vi "Flatness_1.vi"() -> ()   [LabVIEW 2020]
uses:
  Support/Controls/Cmd_Mouse Popup.ctl
  Support/Controls/Clst_Initialize Input.ctl
  Support/Controls/Cmd_Var Data IO.ctl
  Support/Controls/Cmd_STD select.ctl
  Variables/Global_Cal Info.vi
  Variables/Global_Cal STD.vi
panel:
  out "기준기분해능 (μm)":string
  in  "기준기 설정":string(combo)
  in  "Spec 변경":bool
  in  "Random":bool
  out "Spec":string[][](table)
  out "제목":string
  out "에러 출력":errorcluster
  out "Condition":string[][](table) caption="2. 직선성 시험"
  in  "Measured":string[][](table) caption="기준기 지시값 (μm)"
  out "Load?":bool
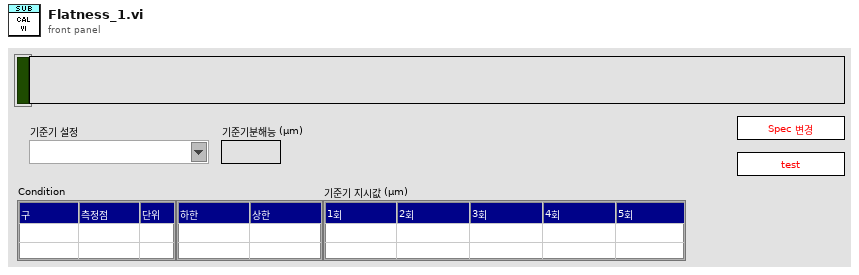
[diagram p1: front panel]
types:
  T1 = typedef "Cmd_Mouse Popup.ctl" = enum16{"활성화", "메뉴선택"}
  T2 = cluster{"Shift":bool, "Ctrl":bool, "Alt":bool, "Cmd":bool, "Opt":bool}
  T3 = typedef "Clst_Initialize Input.ctl" = cluster{"Initialize 1":cluster{"Condition":refnum<vi>[], "Spec":refnum<vi>[], "Measured":refnum<vi>[], "Resolution":refnum<vi>[], "Func_ext":string, "제목":refnum<vi>, "Measured_ADJ":refnum<vi>[]}, "Initialize 2":cluster{"문자열":refnum<vi>[], "콤보박스":refnum<vi>[], "링":refnum<vi>[], "열거형":refnum<vi>[], "테이블":refnum<vi>[], "여러열":refnum<vi>[], "디지털(DBL)":refnum<vi>[], "3D string":refnum<vi>[], "ctrl":refnum<vi>[], "boolean":refnum<vi>[]}}
  T4 = typedef "Cmd_Var Data IO.ctl" = enum16{"Condition", "Condition Default", "Condition_Temp", "Resolution", "Resolution Default", "Resolution Old", "Spec", "Spec Default", "Spec Old", "Spec Temp", "Result", "Result2", "Result3", "Result_Temp", "Result_ADJ", "Result_ADJ2", "STD1", "STD2", "STD3", "STD4", "STD5", "STD Temp", "CMC", "CMC Default"}
  T5 = typedef "Cmd_STD select.ctl" = enum16{"기본", "DMM", "Electronic Micrometer", "Fine Angle Generator", "Measuring Projector", "Precision Square", "Power Supply", "Ring Gauge", "Straight Edge", "Thermo-Hygrometer", "Calibrator"}
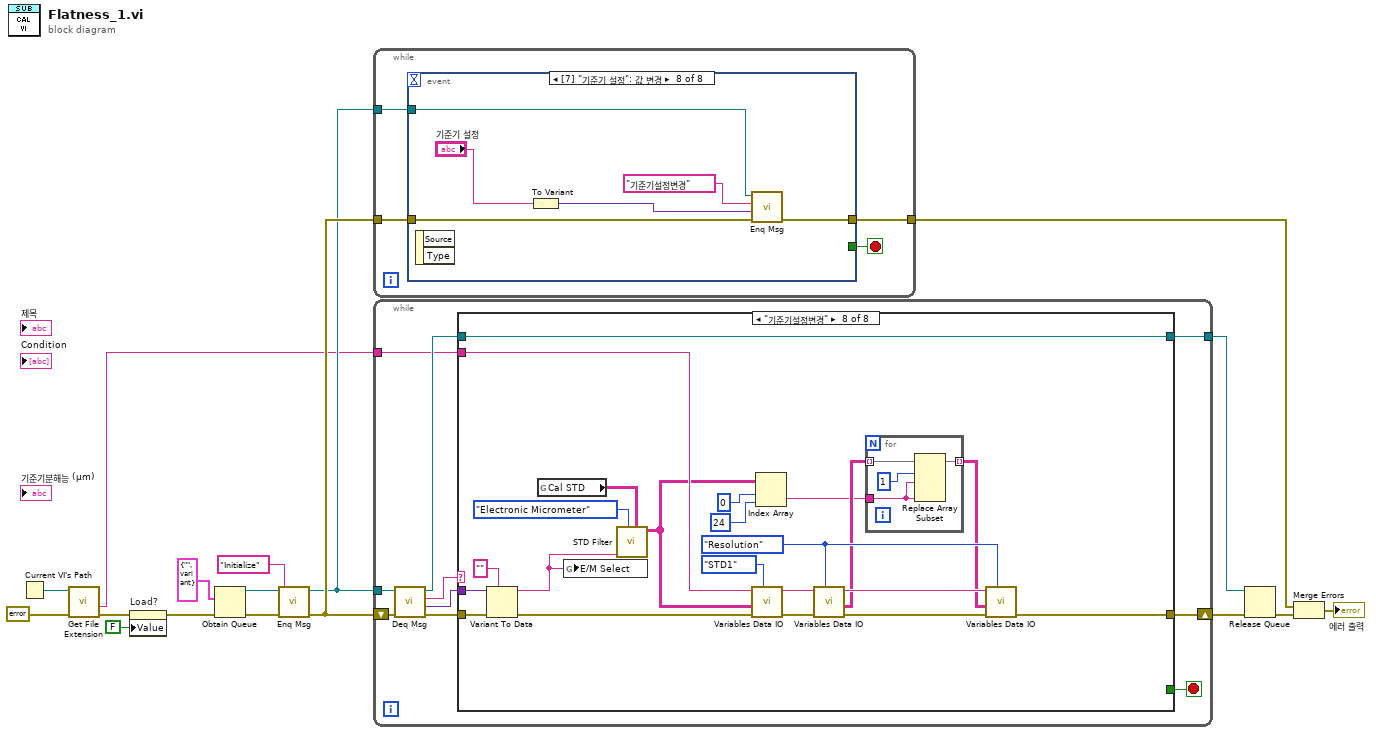
[diagram p0: block diagram]
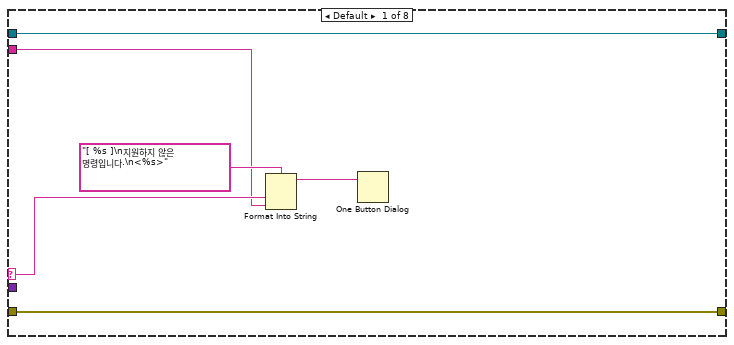
[diagram p2: hidden frame]
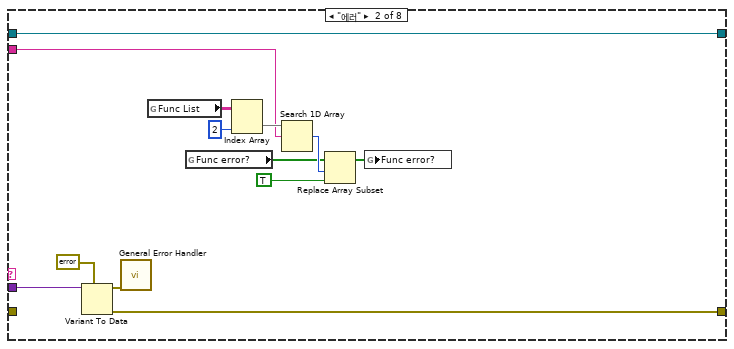
[diagram p3: hidden frame]
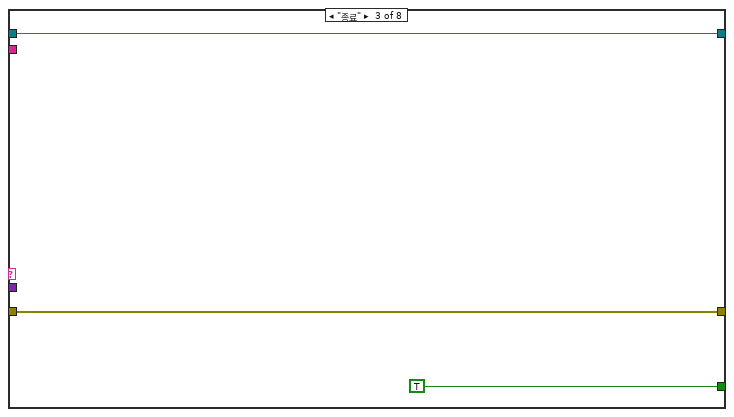
[diagram p4: hidden frame]
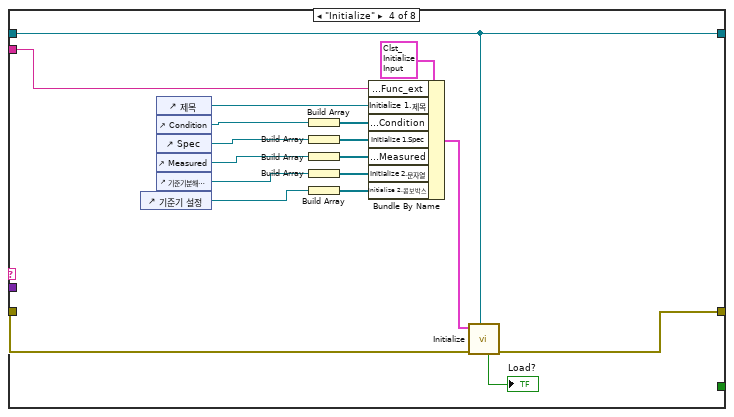
[diagram p5: hidden frame]
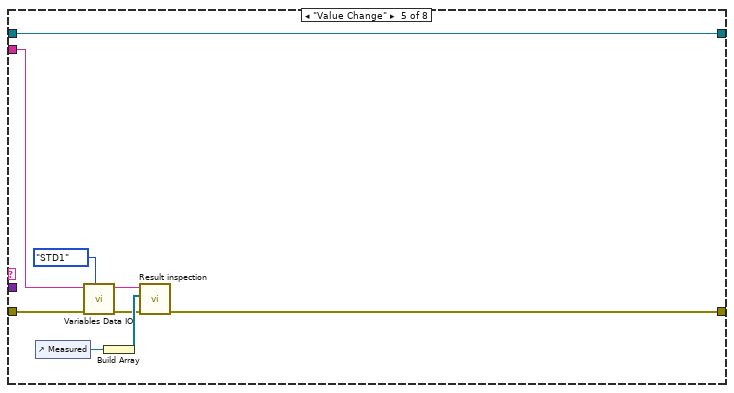
[diagram p6: hidden frame]
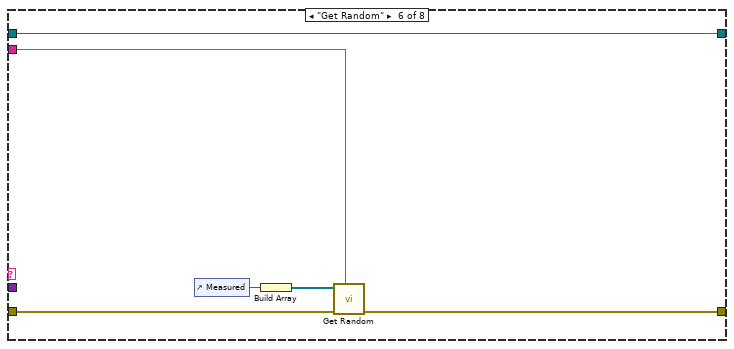
[diagram p7: hidden frame]
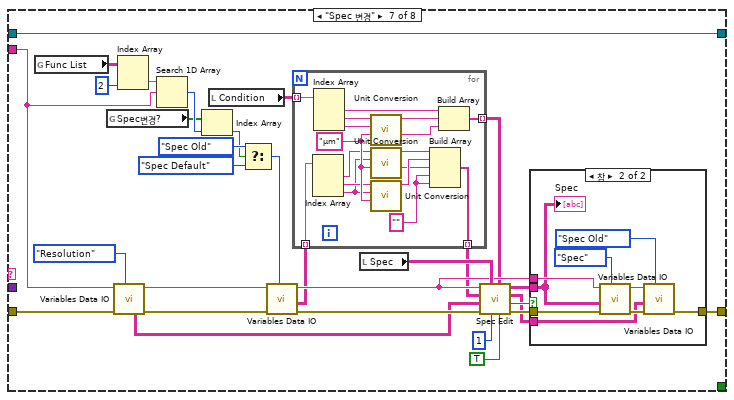
[diagram p8: hidden frame]
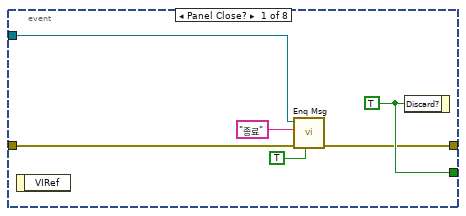
[diagram p10: hidden frame]
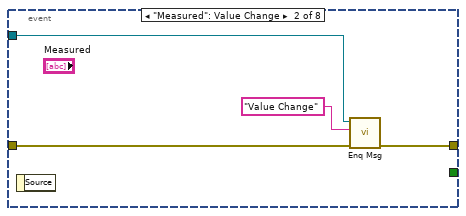
[diagram p11: hidden frame]
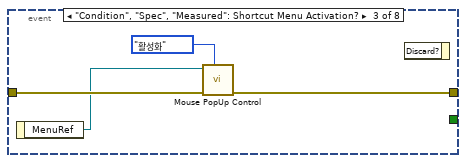
[diagram p12: hidden frame]
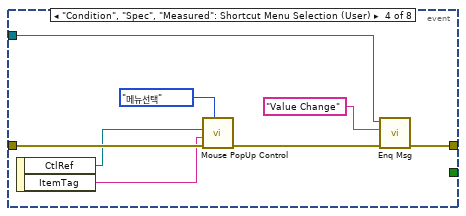
[diagram p13: hidden frame]
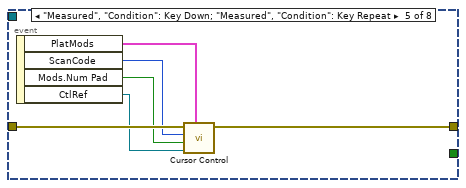
[diagram p14: hidden frame]
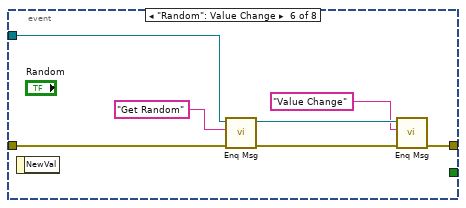
[diagram p15: hidden frame]
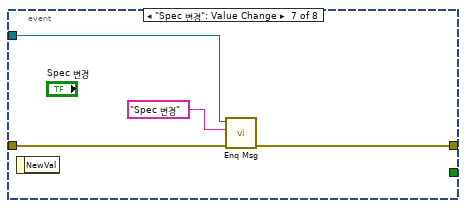
[diagram p16: hidden frame]
diagram:
  n1 = Current VI's Path() -> (path=w5:path)
  n2 = call <vilib>:"Get File Extension.vi"("error in (no error)"=errorcluster {"status"=FALSE, "code"=0, "source"=""} ("에러 상수"), "file"=w5) -> ("error out"=w3:errorcluster, "filename without extension"=w4:string)  [unwired: 5 in, 3 out]
  n3 = property on="Load?" class="Bool (엄격한)"(error in=w3, "Value"=FALSE ("Load?")) -> (error out=w2:errorcluster)  [unwired: 1 in, 1 out]
  n4 = Obtain Queue(element data type=cluster{"메세지":string, "값":variant} {"메세지"="", "값"=variant} ("Message Cluster"), error in (no error)=w2) -> (queue out=w14:refnum<queue>, error out=w16:errorcluster)  [unwired: 3 in, 1 out]
  n5 = call "Enq Msg.vi"("에러 입력(에러 없음)"=w16, "메세지"="Initialize", "큐 입력"=w14) -> ("에러 출력"=w15:errorcluster, "큐 출력"=w12:refnum<queue>)  [unwired: 7 in]
  n6 = while {
    tunnel: w15 -> [w19]
    tunnel: w12 -> [w20]
    tunnel: [w18] -> w9
    stop <- w21 stop-if-true
    n7 = event shown="[7] \"기준기 설정\": 값 변경" {
      selector: _ -> [_ _ _ _ _ _ _ _]
      dyn-events: _ -> [_ _ _ _ _ _ _ _]
      timeout: _ -> [_ _ _ _ _ _ _ _]
      tunnel: [w27 _ _ _ _ _ _ _] -> w21
      tunnel: w20 -> [w25 w31 _ w36 _ w54 w58 w63]
      tunnel: w19 -> [w26 w29 w35 w43 w49 w55 w59 w65]
      tunnel: [w23 w30 w34 w37 w48 w50 w57 w64] -> w18
      event Panel Close? {
        w27 = TRUE ("버림?")
        n8 = event-data() -> ()  [unwired: 1 in, 1 out]
        n9 = call "Enq Msg.vi"("우선순위 메시지?"=TRUE, "에러 입력(에러 없음)"=w26, "메세지"="종료", "큐 입력"=w25) -> ("에러 출력"=w23:errorcluster)  [unwired: 6 in, 1 out]
        n10 = event-data("Discard?"=w27) -> ()  [unwired: 1 in, 1 out]
      }
      event "Measured": Value Change {
        n11 = event-data() -> ()  [unwired: 1 in, 1 out]
        n12 = call "Enq Msg.vi"("에러 입력(에러 없음)"=w29, "메세지"="Value Change", "큐 입력"=w31) -> ("에러 출력"=w30:errorcluster)  [unwired: 7 in, 1 out]
      }
      event "Condition", "Spec", "Measured": Shortcut Menu Activation? {
        n13 = event-data() -> ("MenuRef"=w33:refnum<k9>)  [unwired: 1 in]
        n14 = call "Mouse PopUp Control.vi"("type"=Cmd_Mouse_Popup."활성화", "error in"=w35, "메뉴 참조"=w33) -> ("error out"=w34:errorcluster)  [unwired: 8 in]
        n15 = event-data() -> ()  [unwired: 2 in, 1 out]
      }
      event "Condition", "Spec", "Measured": Shortcut Menu Selection (User) {
        n16 = event-data() -> ("CtlRef"=w41:refnum<vi>, "ItemTag"=w40:string)  [unwired: 1 in]
        n17 = call "Mouse PopUp Control.vi"("type"=Cmd_Mouse_Popup."메뉴선택", "error in"=w43, "아이템 태그"=w40, "Tbl 참조 번호"=w41) -> ("error out"=w38:errorcluster)  [unwired: 7 in]
        n18 = call "Enq Msg.vi"("에러 입력(에러 없음)"=w38, "메세지"="Value Change", "큐 입력"=w36) -> ("에러 출력"=w37:errorcluster)  [unwired: 7 in, 1 out]
      }
      event "Measured", "Condition": Key Down; "Measured", "Condition": Key Repeat {
        n19 = event-data() -> ("PlatMods"=w44:T2, "ScanCode"=w47:i16, "Mods.Num Pad"=w46:bool, "CtlRef"=w45:refnum<vi>)  [unwired: 1 in]
        n20 = call "Cursor Control.vi"("플랫폼 조합키"=w44, "참조"=w45, "Num Pad"=w46, "ScanCode"=w47, "error in"=w49) -> ("error out"=w48:errorcluster)  [unwired: 5 in, 1 out]
      }
      event "Random": Value Change {
        n21 = event-data() -> ()  [unwired: 1 in, 1 out]
        n22 = call "Enq Msg.vi"("에러 입력(에러 없음)"=w55, "메세지"="Get Random", "큐 입력"=w54) -> ("에러 출력"=w53:errorcluster, "큐 출력"=w52:refnum<queue>)  [unwired: 7 in]
        n23 = call "Enq Msg.vi"("에러 입력(에러 없음)"=w53, "메세지"="Value Change", "큐 입력"=w52) -> ("에러 출력"=w50:errorcluster)  [unwired: 7 in, 1 out]
      }
      event "Spec 변경": Value Change {
        n24 = event-data() -> ()  [unwired: 1 in, 1 out]
        n25 = call "Enq Msg.vi"("에러 입력(에러 없음)"=w59, "메세지"="Spec 변경", "큐 입력"=w58) -> ("에러 출력"=w57:errorcluster)  [unwired: 7 in, 1 out]
      }
      event "기준기 설정": Value Change {
        n26 = event-data() -> ()  [unwired: 1 in, 2 out]
        n27 = To Variant(anything="기준기 설정") -> (Variant=w61:variant)
        n28 = call "Enq Msg.vi"("에러 입력(에러 없음)"=w65, "값"=w61, "메세지"="기준기설정변경", "큐 입력"=w63) -> ("에러 출력"=w64:errorcluster)  [unwired: 6 in, 1 out]
      }
    }
  }
  n29 = while {
    shift-right: [w76] -> w11
    shift-left: w15 -> [w75]
    tunnel: w12 -> [w73]
    tunnel: [w68] -> w10
    tunnel: w4 -> [w67]
    stop <- w69 stop-if-true
    n30 = call "Deq Msg.vi"("에러 입력(에러 없음)"=w75, "큐 입력"=w73) -> ("에러 출력"=w74:errorcluster, "값"=w70:variant, "메세지"=w72:string, "큐 출력"=w71:refnum<queue>)  [unwired: 6 in]
    n31 = case shown="\"기준기설정변경\"" w72 {
      selector: w72 -> [w78 _ _ _ _ _ _ _]
      tunnel: w74 -> [w82 _ w98 w116 w120 w127 w154 w209]
      tunnel: [w82 w92 w98 w103 w117 w128 w157 w197] -> w76
      tunnel: w71 -> [w81 w91 w96 w104 w125 w131 w161 w210]
      tunnel: w70 -> [_ w93 _ _ _ _ _ w208]
      tunnel: [_ _ TRUE ("버림?") _ _ _ _ _] -> w69
      tunnel: [w81 w91 w96 w104 w125 w131 w161 w210] -> w68
      tunnel: w67 -> [w77 w83 _ w105 w122 w126 w141 w202]
      frame Default {
        n32 = Format Into String(format string="[ %s ]\n지원하지 않은 명령입니다.\n<%s>" ("메시지"), w78, w77) -> (resulting string=w79:string)  [unwired: 2 in, 1 out]
        n33 = One Button Dialog(message=w79) -> ()  [unwired: 1 in, 1 out]
      }
      frame "에러" {
        n34 = Variant To Data(type=errorcluster {"status"=FALSE, "code"=0, "source"=""} ("에러 출력"), Variant=w93) -> (data=w95:errorcluster, error out=w92:errorcluster)  [unwired: 1 in]
        n35 = call <vilib>:"General Error Handler.vi"("error in (no error)"=w95) -> ()  [unwired: 10 in, 5 out]
        n36 = global read "Global_Cal Info.vi" "Func List"() -> (w85:string[][])
        n37 = global read "Global_Cal Info.vi" "Func error?"() -> (w88:bool[])
        n38 = Index Array(array=w85, index (col)=2 ("비활성화된 인덱스 (열)")) -> (element=w86:string[])  [unwired: 1 in]
        n39 = Search 1D Array(1D array=w86, element=w83) -> (index of element=w89:i32)  [unwired: 1 in]
        n40 = Replace Array Subset(array=w88, new element=TRUE ("새 원소/부분배열"), index=w89) -> (w90:bool[])
        n41 = global write "Global_Cal Info.vi" "Func error?"(w90) -> ()
      }
      frame "종료" {
      }
      frame "Initialize" {
        n42 = control-ref of="기준기 설정"() -> (w100:refnum<vi>)
        n43 = control-ref of="제목"() -> (w108:refnum<vi>)
        n44 = control-ref of="Condition"() -> (w113:refnum<vi>)
        n45 = control-ref of="Spec"() -> (w107:refnum<vi>)
        n46 = control-ref of="Measured"() -> (w110:refnum<vi>)
        n47 = control-ref of="기준기분해능 (μm)"() -> (w99:refnum<vi>)
        n48 = Build Array(w113) -> (w112:refnum<vi>[])
        n49 = Build Array(w107) -> (w106:refnum<vi>[])
        n50 = Build Array(w110) -> (w111:refnum<vi>[])
        n51 = Build Array(w99) -> (w109:refnum<vi>[])
        n52 = Build Array(w100) -> (w101:refnum<vi>[])
        n53 = Bundle By Name(cluster=T3 {"Initialize 1"={"Condition"=[], "Spec"=[], "Measured"=[], "Resolution"=[], "Func_ext"="", "제목"=refnum, "Measured_ADJ"=[]}, "Initialize 2"={"문자열"=[], "콤보박스"=[], "링"=[], "열거형"=[], "테이블"=[], "여러열"=[], "디지털(DBL)"=[], "3D string"=[], "ctrl"=[], "boolean"=[]}} ("입력 클러스터"), "Initialize 1.Func_ext"=w105, "Initialize 1.제목"=w108, "Initialize 1.Condition"=w112, "Initialize 1.Spec"=w106, "Initialize 1.Measured"=w111, "Initialize 2.문자열"=w109, "Initialize 2.콤보박스"=w101) -> (w114:T3)
        n54 = call "Initialize.vi"("큐 입력"=w104, "error in"=w116, "입력 클러스터"=w114) -> ("error out"=w103:errorcluster, "Load?"=→"Load?":bool)  [unwired: 5 in, 2 out]
      }
      frame "Value Change" {
        n55 = control-ref of="Measured"() -> (w124:refnum<vi>)
        n56 = call "Variables Data IO.vi"("Select"=Cmd_Var_Data_IO."STD1", "error in"=w120, "Func_ext"=w122) -> ("error out"=w118:errorcluster, "Func_ext Out"=w119:string)  [unwired: 6 in, 1 out]
        n57 = Build Array(w124) -> (w123:refnum<vi>[])
        n58 = call "Result inspection.vi"("error in"=w118, "Ref. Data (Inspection)"=w123, "Func ext"=w119) -> ("error out"=w117:errorcluster)  [unwired: 5 in, 3 out]
      }
      frame "Get Random" {
        n59 = control-ref of="Measured"() -> (w130:refnum<vi>)
        n60 = Build Array(w130) -> (w129:refnum<vi>[])
        n61 = call "Get Random.vi"("Func_Ext"=w126, "에러 입력"=w127, "Meas"=w129) -> ("에러 출력"=w128:errorcluster)  [unwired: 7 in, 1 out]
      }
      frame "Spec 변경" {
        n62 = global read "Global_Cal Info.vi" "Func List"() -> (w146:string[][])
        n63 = global read "Global_Cal Info.vi" "Spec변경?"() -> (w142:bool[])
        n64 = call "Variables Data IO.vi"("Select"=Cmd_Var_Data_IO."Resolution", "error in"=w154, "Func_ext"=w141) -> ("error out"=w139:errorcluster, "Data Out"=w137:string[][], "Func_ext Out"=w138:string)  [unwired: 6 in]
        n65 = Index Array(array=w146, index (col)=2 ("비활성화된 인덱스 (열)")) -> (element=w144:string[])  [unwired: 1 in]
        n66 = Search 1D Array(1D array=w144, element=w141) -> (index of element=w143:i32)  [unwired: 1 in]
        n67 = Index Array(array=w142, index=w143) -> (element=w147:bool)
        n68 = local read "Condition"() -> (w135:string[][])
        n69 = Select(t=Cmd_Var_Data_IO."Spec Old" ("Select"), s=w147, f=Cmd_Var_Data_IO."Spec Default" ("Select")) -> (s? t:f=w140:T4)
        n70 = call "Variables Data IO.vi"("Select"=w140, "error in"=w139, "Func_ext"=w138) -> ("error out"=w156:errorcluster, "Data Out"=w133:string[][], "Func_ext Out"=w150:string)  [unwired: 6 in]
        n71 = for {
          tunnel: w135 -> [w165] mode=indexing
          tunnel: [w166] -> w134 mode=indexing
          tunnel: w133 -> [w175] mode=indexing
          tunnel: [w168] -> w132 mode=indexing
          w167 = "" ("원소")
          w176 = "μm" ("환산단위")
          n72 = Index Array(array=w175) -> (element #1=w174:string, element #2=w173:string, element #3=w172:string)  [unwired: 3 in]
          n73 = Index Array(array=w165) -> (element #1=w164:string, element #2=w178:string, element #3=w177:string)  [unwired: 3 in]
          n74 = call "Unit Conversion.vi"("환산단위"=w176, "입력단위"=w177, "입력값"=w178) -> ("환산단위"=w162:string, "환산값 (string)"=w163:string)  [unwired: 3 in, 4 out]
          n75 = call "Unit Conversion.vi"("환산단위"=w176, "입력단위"=w172, "입력값"=w174) -> ("환산단위"=w169:string, "환산값 (string)"=w171:string)  [unwired: 3 in, 4 out]
          n76 = call "Unit Conversion.vi"("환산단위"=w176, "입력단위"=w172, "입력값"=w173) -> ("환산값 (string)"=w170:string)  [unwired: 3 in, 5 out]
          n77 = Build Array(w171, w170, w169, w167, w167) -> (w168:string[])
          n78 = Build Array(w164, w163, w162) -> (w166:string[])
        }
        n79 = local read "Spec"() -> (w151:string[][])
        n80 = call "Spec Edit.vi"("0기준?"=TRUE, "Condition"=w134, "열번호(기준값)"=1, "Spec Value"=w151, "에러 입력(에러 없음)"=w156, "Resolution"=w137, "Spec Default"=w132, "Func_ext"=w150) -> ("에러 출력"=w158:errorcluster, "변경?"=w159:bool, "Spec Default out"=w153:string[][], "Spec 출력"=w160:string[][])
        n81 = case shown="참" w159 {
          tunnel: w160 -> [_ w185]
          tunnel: w158 -> [w179 w188]
          tunnel: [w179 w183] -> w157
          tunnel: w150 -> [_ w186]
          tunnel: w153 -> [_ w181]
          frame False {
          }
          frame True {
            n82 = call "Variables Data IO.vi"("Select"=Cmd_Var_Data_IO."Spec", "error in"=w188, "Data In"=w185, "Func_ext"=w186) -> ("error out"=w184:errorcluster, "Func_ext Out"=w182:string)  [unwired: 5 in, 1 out]
            n83 = call "Variables Data IO.vi"("Select"=Cmd_Var_Data_IO."Spec Old", "error in"=w184, "Data In"=w181, "Func_ext"=w182) -> ("error out"=w183:errorcluster)  [unwired: 5 in, 2 out]
            "Spec" <- w185
          }
        }
      }
      frame "기준기설정변경" {
        w195 = Cmd_Var_Data_IO."Resolution" ("Select")
        n84 = Variant To Data(error in=w209, type="", Variant=w208) -> (data=w204:string, error out=w203:errorcluster)
        n85 = global read "Global_Cal STD.vi" "Cal STD"() -> (w205:string[][])
        n86 = global write "Global_Cal STD.vi" "E/M Select"(w204) -> ()
        n87 = call "STD Filter.vi"("Cal STD in"=w205, "STD select"=Cmd_STD_select."Electronic Micrometer", "문자열(option, STD)"=w204) -> ("DATA 출력"=w192:string[][])  [unwired: 4 in, 4 out]
        n88 = call "Variables Data IO.vi"("Select"=Cmd_Var_Data_IO."STD1", "error in"=w203, "Data In"=w192, "Func_ext"=w202) -> ("error out"=w199:errorcluster, "Func_ext Out"=w200:string)  [unwired: 5 in, 1 out]
        n89 = Index Array(array=w192, index (row)=0 ("비활성화된 인덱스 (행)"), index (col)=24 ("비활성화된 인덱스 (열)")) -> (element=w189:string)
        n90 = call "Variables Data IO.vi"("Select"=w195, "error in"=w199, "Func_ext"=w200) -> ("error out"=w198:errorcluster, "Data Out"=w194:string[][], "Func_ext Out"=w196:string)  [unwired: 6 in]
        n91 = for {
          tunnel: w194 -> [w214] mode=indexing
          tunnel: [w213] -> w193 mode=indexing
          tunnel: w189 -> [w212]
          n92 = Replace Array Subset(array=w214, new element #1=w212, index #1=1 ("인덱스"), new element #2=w212) -> (w213:string[])  [unwired: 1 in]
        }
        n93 = call "Variables Data IO.vi"("Select"=w195, "error in"=w198, "Data In"=w193, "Func_ext"=w196) -> ("error out"=w197:errorcluster)  [unwired: 5 in, 2 out]
      }
    }
  }
  n94 = Release Queue(queue=w10, error in (no error)=w11) -> (error out=w8:errorcluster)  [unwired: 1 in, 2 out]
  n95 = Merge Errors(w9, w8) -> (→"에러 출력":errorcluster)
